vi "N-216 Test Panel.vi"() -> ()   [LabVIEW 2016]
uses:
  <vilib>/Instr/_visa.llb/VISA Configure Serial Port (Instr).vi
panel:
  out "USB Settings:Serial Number":string
  out "Error":string
  in  "Check Error":bool
  out "Device Name":string
  out "Response":string
  in  "Quit":bool
  in  "Send Command":bool
  in  "Command":string
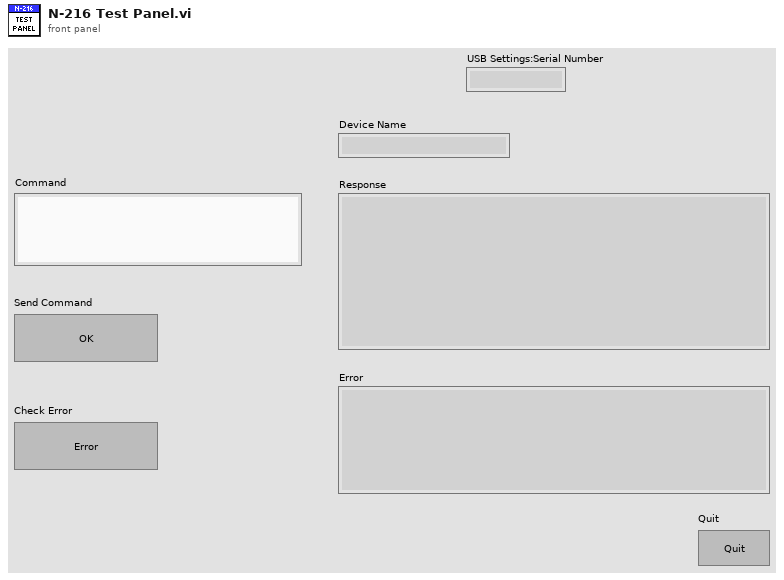
[diagram p1: front panel]
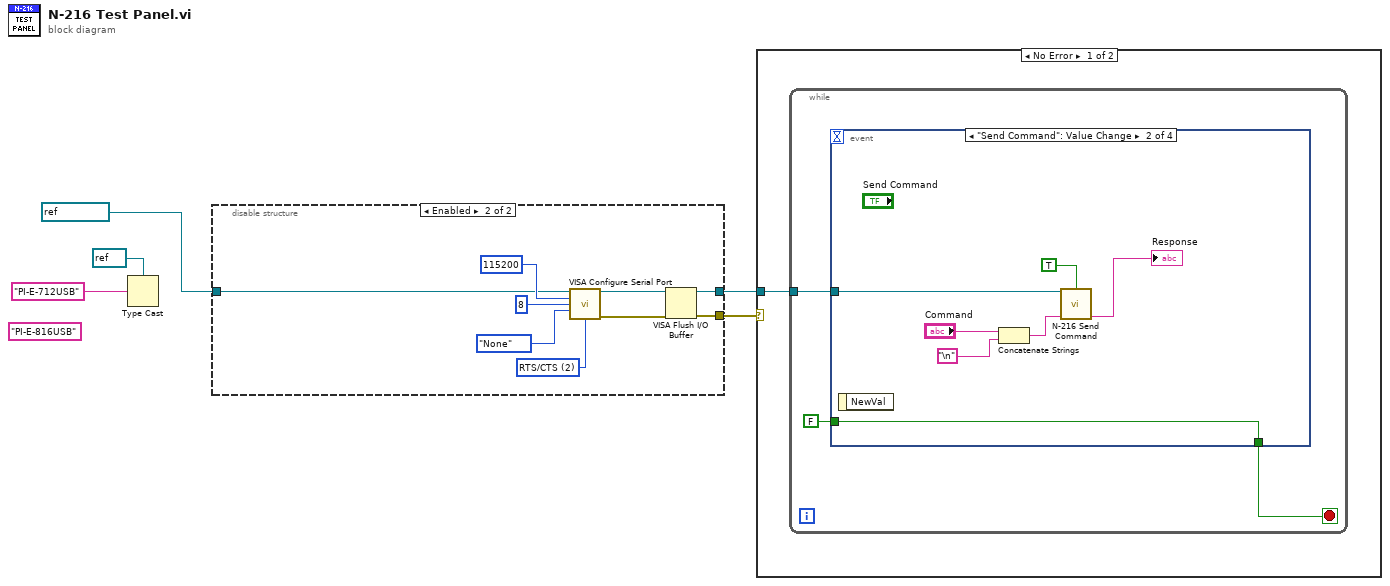
[diagram p0: block diagram]
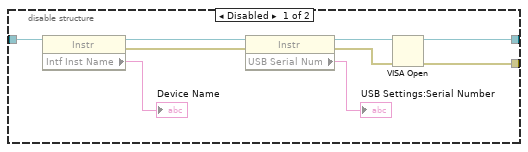
[diagram p2: hidden frame]
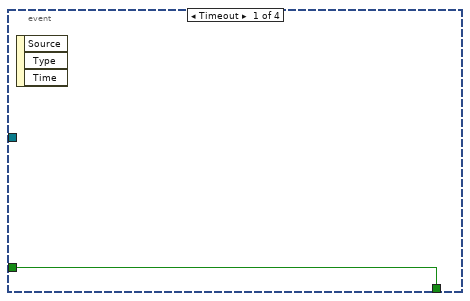
[diagram p3: hidden frame]
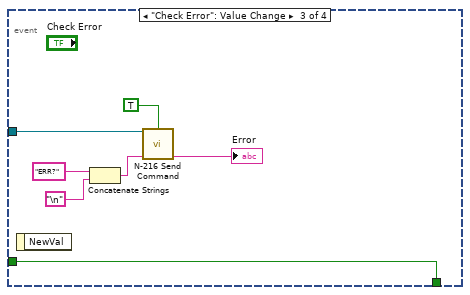
[diagram p4: hidden frame]
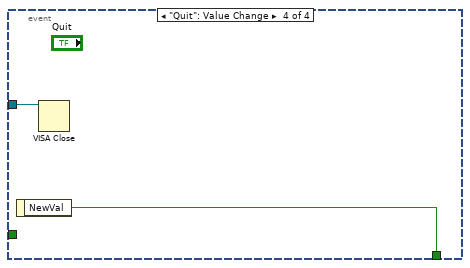
[diagram p5: hidden frame]
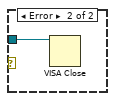
[diagram p6: hidden frame]
diagram:
  (unwired) "PI-E-816USB"
  n1 = Type Cast(type=refnum<visa-resource-name> refnum ("reference out"), x="PI-E-712USB") -> ()  [unwired: 1 out]
  n2 = disable-structure shown="Enabled" {
    disable-tunnel: [w14 w22] -> w5
    disable-tunnel: [w13 w20] -> w3
    disable-tunnel: refnum<visa-resource-name> "COM16" ("reference out") -> [w8 w16]
    frame Disabled {
      n3 = property class="Instr"(reference=w8) -> (reference out=w10:refnum<visa-resource-name>, error out=w12:errorcluster, "Intf Inst Name"=→"Device Name":string)  [unwired: 1 in]
      n4 = property class="Instr"(reference=w10, error in=w12) -> (reference out=w7:refnum<visa-resource-name>, error out=w6:errorcluster, "USB Serial Num"=→"USB Settings:Serial Number":string)
      n5 = VISA Open(error in (no error)=w6, VISA resource name=w7) -> (VISA resource name=w14:refnum<visa-resource-name>, error out=w13:errorcluster)  [unwired: 3 in]
    }
    frame Enabled {
      w15 = u16 2 items=["None", "XON/XOFF", "RTS/CTS", "XON/XOFF & RTS/CTS", "DTR/DSR", "XON/XOFF & DTR/DSR"] ("flow control (0:none)")
      n6 = call-poly "VISA Configure Serial Port"("VISA resource name"=w16, "baud rate (9600)"=u32 115200, "data bits (8)"=u16 8, "parity (0:none)"=enum16{"None", "Odd", "Even", "Mark", "Space"}."None", "flow control (0:none)"=w15) -> ("VISA resource name out"=w23:refnum<visa-resource-name>, "error out"=w21:errorcluster)  [unwired: 9 in]
      n7 = VISA Flush I/O Buffer(VISA resource name=w23, error in (no error)=w21) -> (VISA resource name out=w22:refnum<visa-resource-name>, error out=w20:errorcluster)  [unwired: 1 in]
    }
  }
  n8 = case shown="No Error" w3 {
    tunnel: w5 -> [w24 w45]
    frame No Error {
      n9 = while {
        tunnel: w24 -> [w25]
        stop <- w27 stop-if-true
        n10 = event shown="[1] \"Send Command\": Value Change" {
          selector: _ -> [_ _ _ _]
          dyn-events: _ -> [_ _ _ _]
          timeout: _ -> [_ _ _ _]
          tunnel: [w28 w35 w42 w44] -> w27
          tunnel: FALSE -> [w28 w35 w42 _]
          tunnel: w25 -> [_ w34 w41 w43]
          event Timeout {
            n11 = event-data() -> ()  [unwired: 1 in, 3 out]
          }
          event "Send Command": Value Change {
            n12 = event-data() -> ()  [unwired: 1 in, 1 out]
            n13 = Concatenate Strings("Command", "\n") -> (w29:string)
            n14 = call "N-216 Send Command.vi"("VISA Ref"=w34, "Wait for Reply?"=TRUE, "Command"=w29) -> ("Response"=→"Response":string)  [unwired: 10 in, 2 out]
          }
          event "Check Error": Value Change {
            n15 = event-data() -> ()  [unwired: 1 in, 1 out]
            n16 = Concatenate Strings("ERR?", "\n") -> (w38:string)
            n17 = call "N-216 Send Command.vi"("VISA Ref"=w41, "Wait for Reply?"=TRUE, "Command"=w38) -> ("Response"=→"Error":string)  [unwired: 10 in, 2 out]
          }
          event "Quit": Value Change {
            n18 = event-data() -> ("NewVal"=w44:bool)  [unwired: 1 in]
            n19 = VISA Close(VISA resource name=w43) -> ()  [unwired: 1 in, 1 out]
          }
        }
      }
    }
    frame Error {
      n20 = VISA Close(VISA resource name=w45) -> ()  [unwired: 1 in, 1 out]
    }
  }
